vi "test_looped_handler.vi"() -> ()   [LabVIEW 2025]
uses:
  SLM parameters cluster.ctl
  <userlib>/HOLOEYE SLM Display SDK 4.1.0/types/heds_required_sdk_version_typedef.ctl
  channel parameters cluster.ctl
  <vilib>/Utility/error.llb/DialogType.ctl
  <vilib>/DAQmx/write.llb/DAQmx Write (Analog 1D Wfm NChan NSamp).vi
  <vilib>/DAQmx/write.llb/DAQmx Write (Analog 1D DBL NChan 1Samp).vi
  <vilib>/DAQmx/read.llb/DAQmx Read (Counter U32 1Chan 1Samp).vi
  <vilib>/DAQmx/read.llb/DAQmx Read (Analog Wfm 1Chan NSamp).vi
  <vilib>/Utility/config.llb/Read Key (U32).vi
  <vilib>/Utility/config.llb/Read Key (Path).vi
  <vilib>/DAQmx/miscellaneous.llb/DAQmx Fill In Error Info.vi
  <vilib>/DAQmx/create/channels.llb/DAQmx Create Channel (CI-Count Edges).vi
  <vilib>/DAQmx/configure/trigger.llb/DAQmx Start Trigger (Digital Edge).vi
  <vilib>/DAQmx/create/channels.llb/DAQmx Create Channel (CO-Pulse Generation-Time).vi
  <vilib>/DAQmx/configure/events/hardwareSignals.llb/DAQmx Export Signal (Most Signals).vi
  <resource>/dialog/BookmarkManager/managers/Default/support/User Event - Stop/BMark_User Event - Stop.lvlib
  <vilib>/Utility/config.llb/NI_LVConfig.lvlib
  <resource>/objmgr/daqmx.rc
panel:
  out "Trial progess slide":u8(slide) caption="trials" scale=0.0..5.0
  in  "Acquire time block":bool
  out "SLM image":picture
  in  "File prefix":string
  in  "Begin Experiment":bool caption="Begin experiment"
  in  "Save directory":path=path "D:/KinetixTest/SS_test"
  in  "# Trials":u32=1 caption="trials" min=1 step=1
  in  "Trial Time":dbl=1.0 caption="s" min=0.1 max=60.0 format="%#_2g"
  in  "slow camera frequency":u16(ring)=10 caption="Hz" items=["10"=10, "20"=20, "50"=50]
  in  "scan/fast camera frequency":u16(ring)=100 caption="Hz" items=["20"=20, "100"=100, "800"=800]
  in  "Pulse Duty Cycle":dbl=50.0 caption="%" min=1.0 max=100.0 step=0.1
  in  "Pulse 470":bool
  in  "Dichroic/dual imaging":bool
  out "SLM connected":bool
  in  "Connect SLM":bool
  in  "SLM default":bool
  in  "Load SLM image":bool
  in  "Create SLM image":bool
  in  "470 nm LED control":dbl(slide) step=1.0 scale=0.0..100.0 scale format="%#_3g"
  in  "594 nm laser control":dbl(slide) step=1.0 scale=0.0..100.0 scale format="%#_3g"
  in  "Run time":i32 caption="s" min=0
  in  "Run Live":bool caption="Run live"
  in  "Galvo voltage":dbl=1.0 caption="V" min=0.1 max=1.8 format="%#_2g"
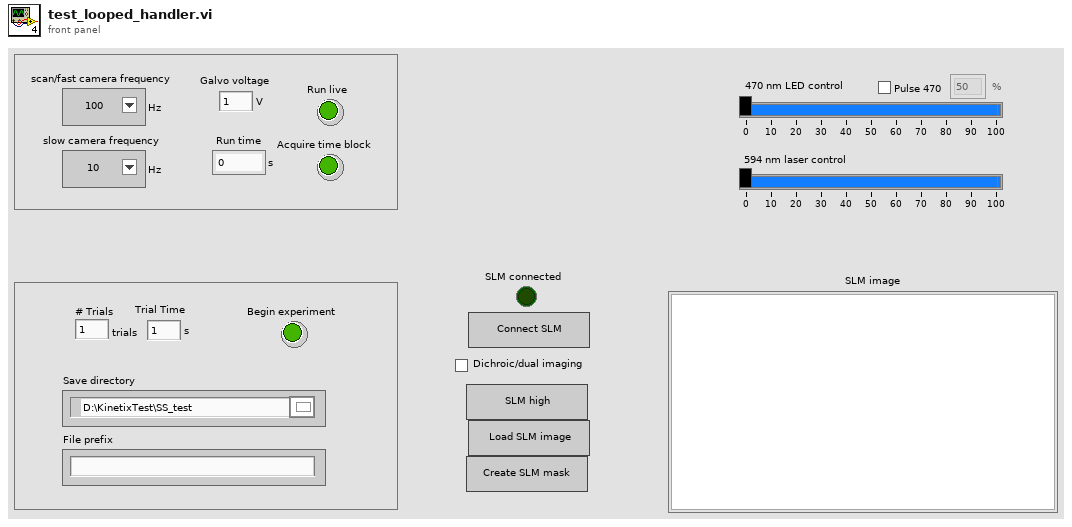
[diagram p1: front panel]
types:
  T1 = typedef "All Message Queues_TICO behavior.ctl" = cluster{"DAQ":refnum<queue>, "Acquisition":refnum<queue>, "Kinetix":refnum<queue>, "ThorCam":refnum<queue>, "SLM":refnum<queue>, "stop":refnum<queue>, " UI":refnum<queue>}
  T2 = typedef "SLM parameters cluster.ctl" = cluster{"SLM cols":u32, "SLM rows":u32, " camera image rows":u32, "camera image cols":u32, "high image (no DM)":path, "low image (no DM)":path, "high image (DM)":path, "low image (DM)":path}
  T3 = typedef "heds_required_sdk_version_typedef.ctl" = cluster{"Major Version Number":i32, "Minor Version Number":i32}
  T4 = typedef "NI_LVConfig.lvlib/Config Data RefNum.ctl" = refnum<k1>
  T5 = typedef "heds_slm_id_typedef.ctl" = cluster{"slmwindow_id":u32, "slmscreen_id":u32}
  T6 = enum8{"Enabled", "Disabled", "Disabled and Grayed Out"}
  T7 = typedef "IMAQ Image.ctl" = refnum<image>
  T8 = typedef "channel parameters cluster.ctl" = cluster{"voltage":dbl, "frequency":dbl, "duty cycle":dbl, "sample rate":dbl}
  T9 = cluster{"shutter trigger":refnum<k21>, "galvo control":refnum<k21>, "Kinetix trigger":refnum<k21>, "Kinetix readout":refnum<k21>, "Zelux trigger":refnum<k21>, "Zelux readout":refnum<k21>}
  T10 = typedef "DialogType.ctl" = u16
  T11 = enum16{"open", "open or create", "create or replace", "create", "open (read-only)"}
  T12 = typedef "Camera Description.ctl" = cluster{"Serial Number":string, "Chip Name":string, "Sensor Width":u32, "Sensor Height":u32, "Firmware version":string, "Interface":string, "Part Number":string, "Product Name":string}
  T13 = cluster{"Camera 0 Name ":string, "Camera Description":T12}
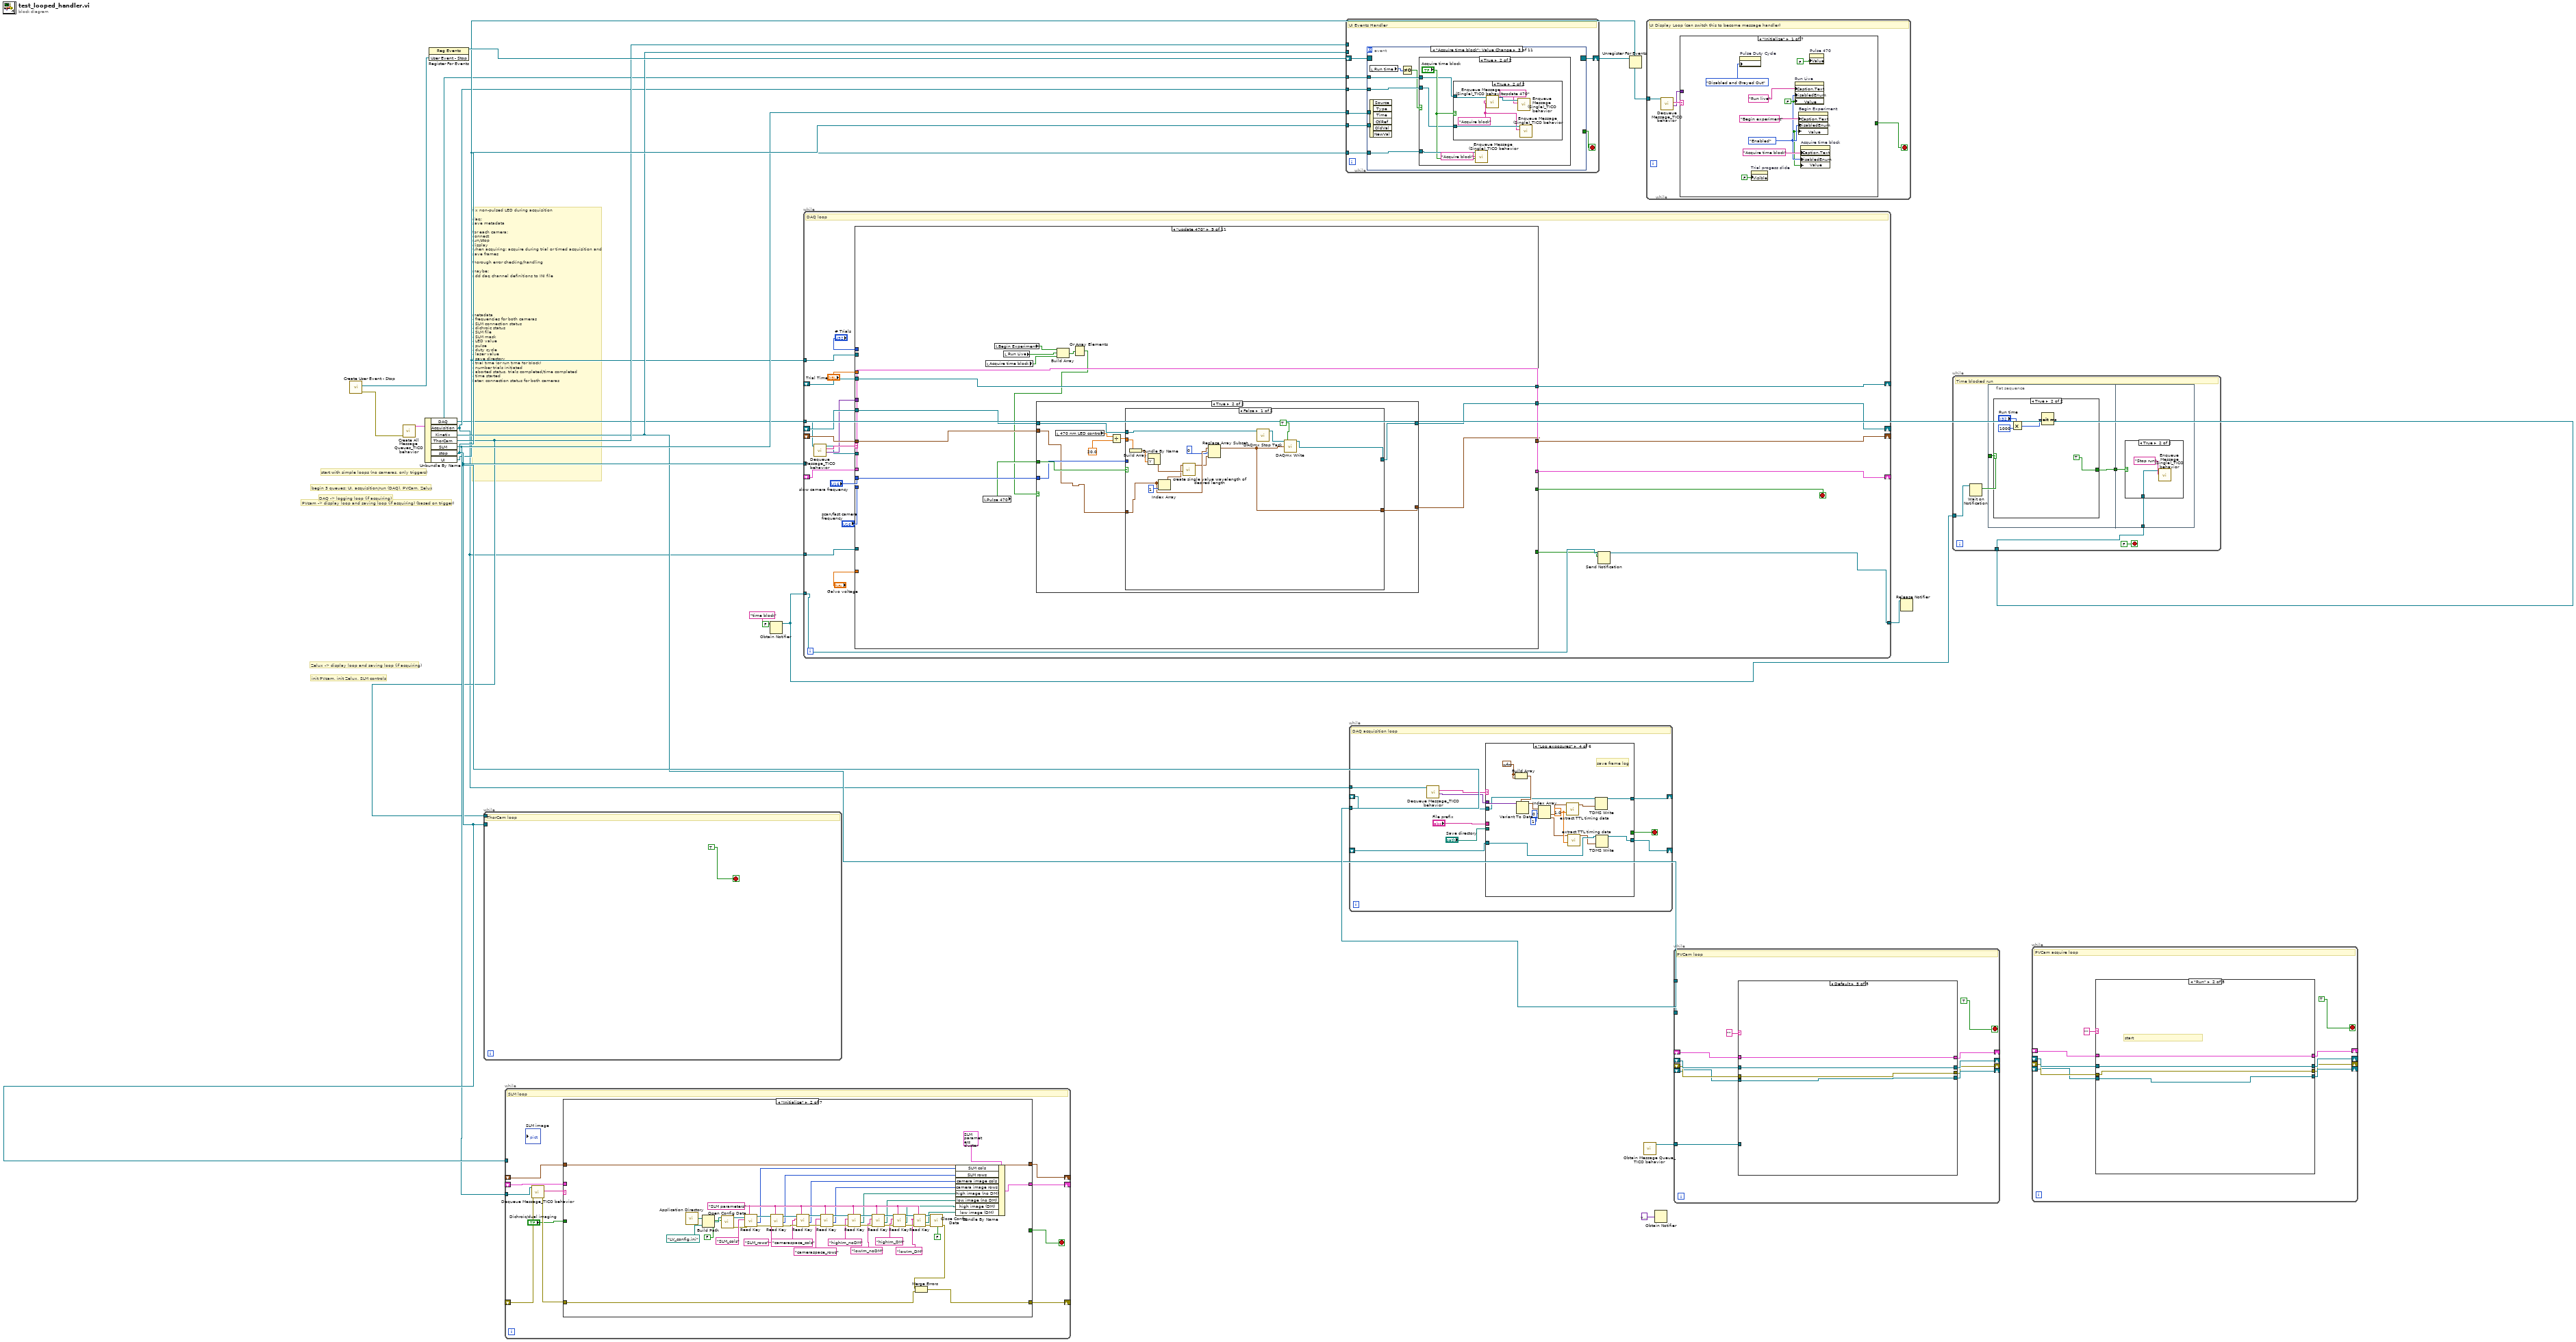
[diagram p0: block diagram]
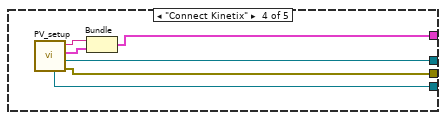
[diagram p4: hidden frame]
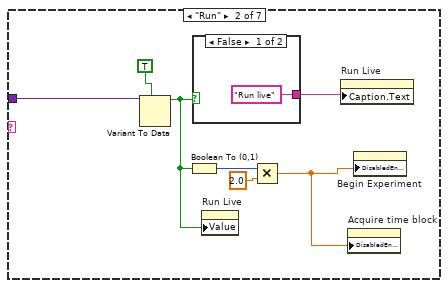
[diagram p8: hidden frame]
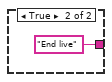
[diagram p9: hidden frame]
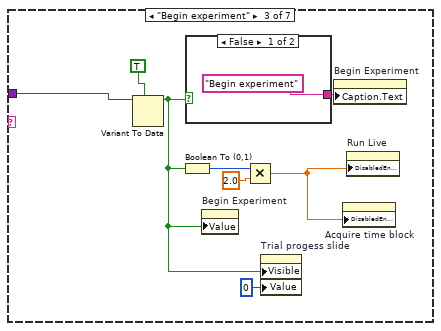
[diagram p10: hidden frame]
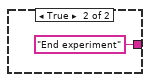
[diagram p11: hidden frame]
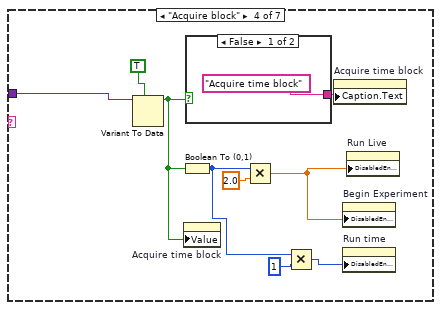
[diagram p12: hidden frame]
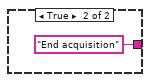
[diagram p13: hidden frame]
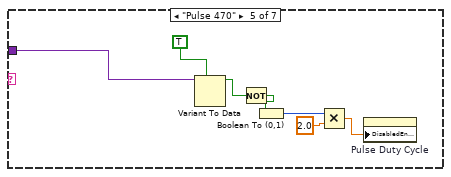
[diagram p14: hidden frame]
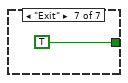
[diagram p16: hidden frame]
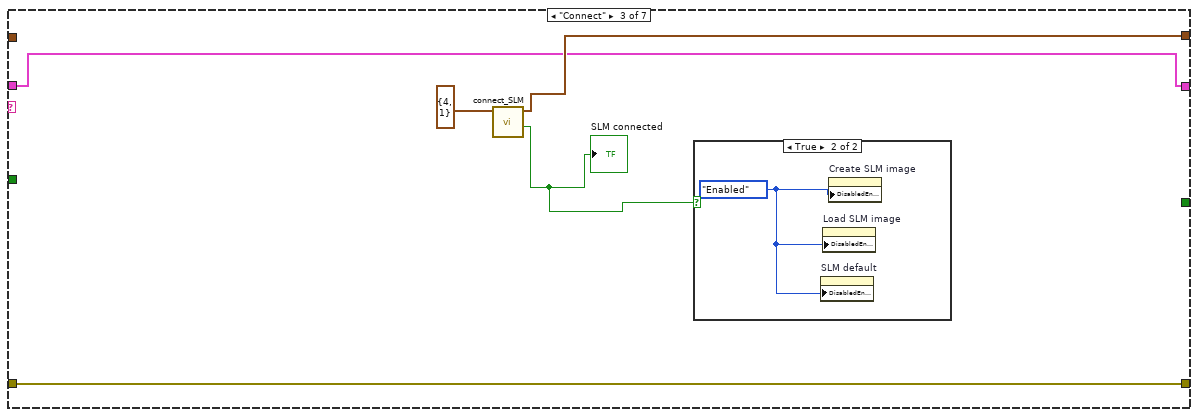
[diagram p18: hidden frame]
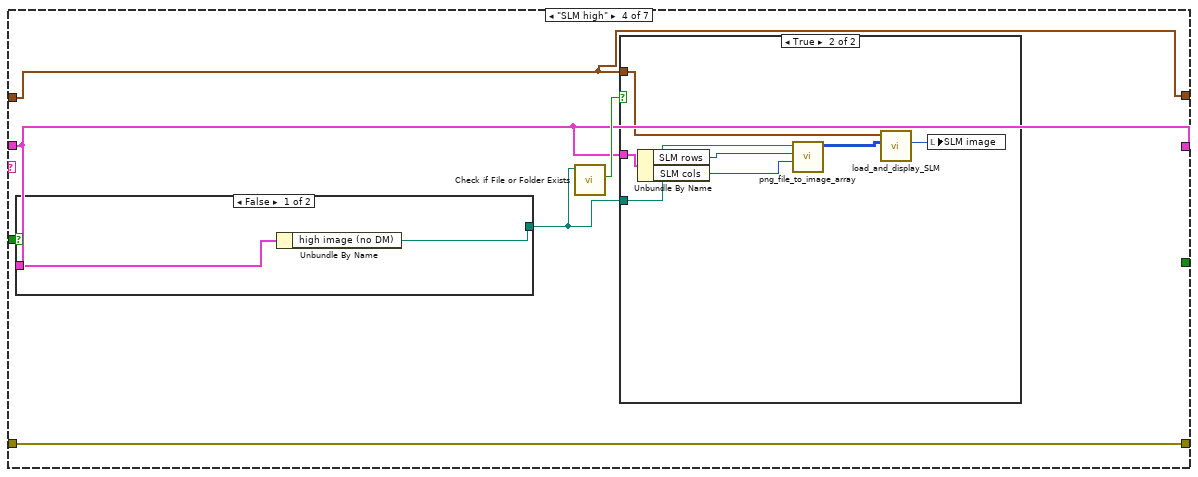
[diagram p20: hidden frame]
diagram:
  # "fix non-pulsed LED during acquisition\n\ndaq:\nsave metadata\n\nfor each camera:\nconnect\nrun/stop\ndisplay\nwhen acquiring: acquire during trial or timed acquisition and \nsave frames\n\nthorough error checking/handling\n\nmaybe:\nadd daq channel definitions to INI file\n\n\n\n\n\n\n\n\nmetadata\n- frequencies for both cameras\n- SLM connection status\n- dichroic status\n- SLM file\n- SLM mask\n- LED value\n- pulse\n- duty cycle\n- laser value\n- save directory\n- trial time (or run time for block)\n- number trials initiated\n- aborted status, trials completed/time completed \n- time started\nLater: connection status for both cameras"
  # "start with simple loops (no cameras, only triggers)"
  # "init PVcam, init Zelux, SLM controls"
  # "Zelux -> display loop and saving loop (if acquiring)"
  # "PVcam -> display loop and saving loop (if acquiring) (based on trigger)"
  # "DAQ -> logging loop (if acquiring)"
  # "begin 3 queues: UI, acquisition/run (DAQ), PVCam, Zelux"
  n1 = call <resource>:"Create User Event - Stop.vi"() -> ("error out"=w17:errorcluster, "User Event - Stop"=w16:refnum<user-event>)  [unwired: 10 in]
  n2 = call "Create All Message Queues_TICO behavior.vi"("error in (no error)"=w17) -> ("Message Queues out"=w18:T1)  [unwired: 9 in, 1 out]
  n3 = Unbundle By Name(w18) -> ("DAQ"=w3:refnum<queue>, "Acquisition"=w4:refnum<queue>, "Kinetix"=w10:refnum<queue>, "ThorCam"=w11:refnum<queue>, "SLM"=w12:refnum<queue>, "stop"=w13:refnum<queue>, "UI"=w9:refnum<queue>)
  n4 = register-events(w16) -> (reference out=w15:refnum<event-registration>)  [unwired: 2 in, 1 out]
  n5 = while {
    tunnel: w11 -> [_]
    tunnel: w13 -> [_]
    stop <- TRUE stop-if-true
    # "ThorCam loop"
  }
  n6 = while {
    tunnel: w12 -> [w27]
    tunnel: w13 -> [_]
    shift-right: [w29] -> _
    shift-left: _ -> [w28]
    shift-right: [w24] -> _
    shift-left: _ -> [w26]
    shift-right: [w22] -> _
    shift-left: _ -> [w21]
    stop <- w23 stop-if-true
    # "SLM loop"
    n7 = call "Dequeue Message_TICO behavior.vi"("error in (no error)"=w26, "Message Queue"=w27) -> ("error out"=w25:errorcluster, "Message"=w30:string)  [unwired: 6 in, 2 out]
    n8 = case shown="\"Initialize\"" w30 {
      tunnel: [w31 w79 w82 w88 w109 w123 w163] -> w29
      tunnel: w28 -> [w31 w79 _ w88 w109 w123 w163]
      tunnel: w25 -> [w32 w70 w81 w91 w108 w120 w162]
      tunnel: [w32 w71 w81 w91 w108 w120 w161] -> w24
      tunnel: [_ _ _ _ _ _ TRUE] -> w23
      tunnel: [w33 w34 w80 w86 w110 w119 w160] -> w22
      tunnel: w21 -> [w33 _ w80 w86 w110 w119 w160]
      tunnel: "Dichroic/dual imaging" -> [_ _ _ w87 _ w137 _]
      frame Default {
      }
      frame "Initialize" {
        w60 = "SLM parameters" ("section")
        n9 = call <vilib>:"Application Directory.vi"() -> ("Application Directory"=w77:path)
        n10 = Build Path(base path=w77, name or relative path=path "LV_config.ini" ("default name")) -> (appended path=w76:path)
        n11 = call <vilib>:"Open Config Data.vi"("create file if necessary (T)"=FALSE, "configuration file path"=w76) -> ("error out"=w72:errorcluster, "refnum"=w74:T4)  [unwired: 7 in, 1 out]
        n12 = call-poly <vilib>:"Read Key.vi"("section"=w60, "error in (no error)"=w72, "key"="SLM_cols", "refnum"=w74) -> ("error out"=w69:errorcluster, "value"=w42:u32, "refnum out"=w68:T4)  [unwired: 4 in, 1 out]
        n13 = call-poly <vilib>:"Read Key.vi"("section"=w60, "error in (no error)"=w69, "key"="SLM_rows", "refnum"=w68) -> ("error out"=w61:errorcluster, "value"=w41:u32, "refnum out"=w59:T4)  [unwired: 4 in, 1 out]
        n14 = call-poly <vilib>:"Read Key.vi"("section"=w60, "error in (no error)"=w61, "key"="cameraspace_cols", "refnum"=w59) -> ("error out"=w62:errorcluster, "value"=w40:u32, "refnum out"=w58:T4)  [unwired: 4 in, 1 out]
        n15 = call-poly <vilib>:"Read Key.vi"("section"=w60, "error in (no error)"=w62, "key"="cameraspace_rows", "refnum"=w58) -> ("error out"=w63:errorcluster, "value"=w39:u32, "refnum out"=w57:T4)  [unwired: 4 in, 1 out]
        n16 = call-poly <vilib>:"Read Key.vi"("section"=w60, "error in (no error)"=w63, "key"="highIm_noDM", "refnum"=w57) -> ("error out"=w64:errorcluster, "value"=w38:path, "refnum out"=w56:T4)  [unwired: 4 in, 1 out]
        n17 = call-poly <vilib>:"Read Key.vi"("section"=w60, "error in (no error)"=w64, "key"="lowIm_noDM", "refnum"=w56) -> ("error out"=w65:errorcluster, "value"=w37:path, "refnum out"=w55:T4)  [unwired: 4 in, 1 out]
        n18 = call-poly <vilib>:"Read Key.vi"("section"=w60, "error in (no error)"=w65, "key"="highIm_DM", "refnum"=w55) -> ("error out"=w66:errorcluster, "value"=w36:path, "refnum out"=w54:T4)  [unwired: 4 in, 1 out]
        n19 = call-poly <vilib>:"Read Key.vi"("section"=w60, "error in (no error)"=w66, "key"="lowIm_DM", "refnum"=w54) -> ("error out"=w53:errorcluster, "value"=w35:path, "refnum out"=w52:T4)  [unwired: 4 in, 1 out]
        n20 = call <vilib>:"Close Config Data.vi"("error in (no error)"=w53, "write file if changed (T)"=FALSE, "refnum"=w52) -> ("error out"=w50:errorcluster)  [unwired: 8 out]
        n21 = Merge Errors(w50, w70) -> (w71:errorcluster)
        n22 = Bundle By Name(cluster=T2 {"SLM cols"=0, "SLM rows"=0, " camera image rows"=0, "camera image cols"=0, "high image (no DM)"=path "", "low image (no DM)"=path "", "high image (DM)"=path "", "low image (DM)"=path ""} ("input cluster"), "SLM cols"=w42, "SLM rows"=w41, "camera image cols"=w40, "camera image rows"=w39, "high image (no DM)"=w38, "low image (no DM)"=w37, "high image (DM)"=w36, "low image (DM)"=w35) -> (w34:T2)
      }
      frame "Connect" {
        n23 = call "connect_SLM.vi"("Required SDK version"=T3 {"Major Version Number"=4, "Minor Version Number"=1}) -> ("SLM connected"=w83:bool, "SLM ID"=w82:T5)  [unwired: 9 in]
        "SLM connected" <- w83
        n24 = case shown="True" w83 {
          frame False {
          }
          frame True {
            w85 = T6."Enabled" ("Disabled")
            n25 = property on="SLM default" class="Bool"("DisabledEnum"=w85) -> ()  [unwired: 2 in, 2 out]
            n26 = property on="Load SLM image" class="Bool"("DisabledEnum"=w85) -> ()  [unwired: 2 in, 2 out]
            n27 = property on="Create SLM image" class="Bool"("DisabledEnum"=w85) -> ()  [unwired: 2 in, 2 out]
          }
        }
      }
      frame "SLM high" {
        n28 = case shown="False" w87 {
          tunnel: [w92 w94] -> w90
          tunnel: w86 -> [w93 w95]
          frame False {
            n29 = Unbundle By Name(w93) -> ("high image (no DM)"=w92:path)
          }
          frame True {
            n30 = Unbundle By Name(w95) -> ("high image (DM)"=w94:path)
          }
        }
        n31 = call <vilib>:"Check if File or Folder Exists.vi"("path"=w90) -> ("file or folder exists?"=w89:bool)  [unwired: 8 in, 2 out]
        n32 = case shown="True" w89 {
          tunnel: w90 -> [_ w102]
          tunnel: w88 -> [_ w99]
          tunnel: w86 -> [_ w98]
          frame False {
          }
          frame True {
            n33 = Unbundle By Name(w98) -> ("SLM rows"=w97:u32, "SLM cols"=w96:u32)
            n34 = call "png_file_to_image_array.vi"("dimension size 2"=w96, "dimension size 1"=w97, "path to PNG file"=w102) -> ("output array"=w101:u8[][])  [unwired: 8 in]
            n35 = call "load_and_display_SLM.vi"("Image Data"=w101, "SLM ID"=w99) -> ("2D Picture"=w100:picture)  [unwired: 8 in, 1 out]
            n36 = local write "SLM image"(w100) -> ()
          }
        }
      }
      frame "Load image" {
        n37 = local read "Save directory"() -> (w107:path)
        n38 = call "IMAQ Load Image Dialog"("Pattern"="SLM_pattern_*.png*" ("pattern (all files)"), "Multiple Files? (No)"=FALSE, "Start Path"=w107) -> ("Path"=w104:path)  [unwired: 6 in, 2 out]
        n39 = call <vilib>:"Check if File or Folder Exists.vi"("path"=w104) -> ("file or folder exists?"=w111:bool, "dup path"=w103:path)  [unwired: 8 in, 1 out]
        n40 = case shown="True" w111 {
          tunnel: w109 -> [_ w117]
          tunnel: w110 -> [_ w116]
          tunnel: w103 -> [_ w112]
          frame False {
          }
          frame True {
            n41 = Unbundle By Name(w116) -> ("SLM rows"=w115:u32, "SLM cols"=w114:u32)
            n42 = call "png_file_to_image_array.vi"("dimension size 2"=w114, "dimension size 1"=w115, "path to PNG file"=w112) -> ("output array"=w118:u8[][])  [unwired: 8 in]
            n43 = call "load_and_display_SLM.vi"("Image Data"=w118, "SLM ID"=w117) -> ("2D Picture"=w113:picture)  [unwired: 8 in, 1 out]
            n44 = local write "SLM image"(w113) -> ()
          }
        }
      }
      frame "Create mask" {
        n45 = local read "Save directory"() -> (w152:path)
        n46 = Unbundle By Name(w119) -> ("camera image rows"=w143:u32, "camera image cols"=w142:u32, "SLM rows"=w139:u32, "SLM cols"=w140:u32)
        n47 = call "IMAQ Load Image Dialog"("Pattern"="*.tif*" ("pattern (all files)"), "Multiple Files? (No)"=FALSE, "Start Path"=w152) -> ("Path"=w153:path)  [unwired: 6 in, 2 out]
        n48 = call "create ROIs GUI.vi"("Mask high value (default 255)"=sgl 255.0, "TIFF path"=w153) -> ("error out"=w148:errorcluster, "ROI mask image"=w147:T7)  [unwired: 8 in]
        n49 = case shown="False" w137 {
          tunnel: w119 -> [w156 w159]
          tunnel: [w155 w158] -> w136
          tunnel: [w154 w157] -> w135
          frame False {
            n50 = Unbundle By Name(w156) -> ("high image (no DM)"=w155:path, "low image (no DM)"=w154:path)
          }
          frame True {
            n51 = Unbundle By Name(w159) -> ("high image (DM)"=w158:path, "low image (DM)"=w157:path)
          }
        }
        n52 = call "IMAQ GetImageSize"("Image"=w147) -> ("Y Resolution"=w145:i32, "X Resolution"=w146:i32)  [unwired: 3 in, 1 out]
        n53 = call "crop_image_to_SLM_size.vi"("Y max"=w142, "X max"=w143, "error in (no error)"=w148, "Y size"=w145, "X size"=w146, "Image Src"=w147) -> ("error out"=w141:errorcluster, "Image Dst Out"=w144:T7)  [unwired: 4 in]
        n54 = call "resize camera space image to SLM space.vi"("Y SLM"=w139, "X SLM"=w140, "error in (no error)"=w141, "Y camera"=w142, "X camera"=w143, "original image"=w144) -> ("Resized image"=w138:T7)  [unwired: 4 in, 1 out]
        n55 = call "create SLM image from mask.vi"("low image path"=w135, "high image path"=w136, "Mask"=w138) -> ("Image Pixels (U8)"=w124:u8[][], "Final image"=w126:T7)  [unwired: 7 in]
        n56 = local read "File prefix"() -> (w121:string)
        n57 = local read "Save directory"() -> (w122:path)
        n58 = Format Date/Time String(time format string (%c)="%Y%m%d_%H%M%S.png") -> (date/time string=w134:string)  [unwired: 2 in]
        n59 = Concatenate Strings("SLM_pattern_" ("string"), w121, w134) -> (w133:string)
        n60 = call "load_and_display_SLM.vi"("Image Data"=w124, "SLM ID"=w123) -> ("2D Picture"=w125:picture)  [unwired: 8 in, 1 out]
        n61 = String To Path(string=w133) -> (path=w132:path)
        n62 = local write "SLM image"(w125) -> ()
        n63 = Build Path(base path=w122, name or relative path=w132) -> (appended path=w131:path)
        n64 = call-poly "IMAQ Write File 2"("Use bit depth? (false)"=TRUE, "Image Quality"=u32 1000, "File Path"=w131, "Image"=w126) -> ()  [unwired: 6 in, 2 out]
      }
      frame "Stop" {
        n65 = call <userlib>:"heds_close.vi"("error in (no error)"=w162) -> ("error out"=w161:errorcluster)  [unwired: 10 in]
      }
    }
  }
  n66 = Obtain Notifier(name (unnamed)="time block", notification data type=FALSE) -> (notifier out=w6:refnum<notifier>)  [unwired: 2 in, 2 out]
  n67 = while {
    tunnel: w3 -> [w170]
    tunnel: w13 -> [_]
    shift-right: [w184] -> _
    shift-left: _ -> [w183]
    shift-right: [w182] -> _
    shift-left: _ -> [w181]
    shift-right: [w180] -> _
    shift-left: _ -> [w179]
    tunnel: w9 -> [w176]
    tunnel: w6 -> [w174]
    tunnel: [w175] -> w7
    shift-right: [w172] -> _
    shift-left: _ -> [w171]
    tunnel: w4 -> [w168]
    stop <- w178 stop-if-true
    # "DAQ loop"
    n68 = call "Dequeue Message_TICO behavior.vi"("Message Queue"=w170) -> ("Message Data"=w166:variant, "Message"=w187:string, "dup Message Queue"=w165:refnum<queue>)  [unwired: 7 in, 1 out]
    n69 = case shown="\"update 470\"" w187 {
      selector: w187 -> [_ _ _ w264 _ _ _ _ _ _ _]
      tunnel: "scan/fast camera frequency" -> [_ w222 _ w336 _ _ _ _ _ _ _]
      tunnel: "slow camera frequency" -> [_ w223 _ w335 _ _ _ _ w513 _ _]
      tunnel: [w198 w205 w236 w332 w374 w423 w489 w499 w515 w566 w571] -> w184
      tunnel: w183 -> [_ w205 w255 w279 w374 w422 w489 w500 w516 w566 w571]
      tunnel: [w189 w224 w226 w334 w375 w416 w488 w491 w512 w565 w570] -> w182
      tunnel: w181 -> [_ w224 w229 w334 w375 w413 w488 w494 w514 w565 w570]
      tunnel: [w201 w220 T9 {"shutter trigger"="", "galvo control"="", "Kinetix trigger"="", "Kinetix readout"="", "Zelux trigger"="", "Zelux readout"=""} ("tasks cluster") w283 w372 T9 {"shutter trigger"="", "galvo control"="", "Kinetix trigger"="", "Kinetix readout"="", "Zelux trigger"="", "Zelux readout"=""} ("tasks cluster") w463 w502 w517 w564 w569] -> w180
      tunnel: w179 -> [w201 _ w254 _ w373 w457 w464 w502 w517 w564 w569]
      tunnel: [_ _ FALSE _ _ _ _ _ _ _ TRUE] -> w178
      tunnel: "Galvo voltage" -> [_ w209 _ w297 _ _ _ _ _ _ _]
      tunnel: [_ w203 _ _ _ _ _ _ _ _ _] -> w167
      tunnel: w176 -> [_ _ w232 _ _ w408 _ _ _ _ _]
      tunnel: "Trial Time" -> [_ _ _ w266 w368 _ _ _ _ _ _]
      tunnel: [w188 w202 refnum<k21> refnum ("task out") w282 w363 refnum<k21> refnum ("task out") w465 w490 w510 w563 w567] -> w172
      tunnel: w171 -> [w188 w202 _ _ w382 w431 w465 w490 w510 w563 w567]
      tunnel: w165 -> [_ _ _ w263 w381 w403 w487 _ _ _ _]
      tunnel: "# Trials" -> [_ _ _ w258 w362 _ _ _ _ _ _]
      tunnel: w168 -> [_ _ _ w281 w378 w430 _ _ _ _ _]
      tunnel: w166 -> [_ _ _ _ w364 _ _ _ _ _ _]
      frame "Initialize" {
        # "start tasks for LED and laser"
        n70 = call "init_lasers.vi"("488 pulsed"=FALSE, "594 nm voltage"=0.0, "488 nm channel parameters"=T8 {"voltage"=0.0, "frequency"=0.0, "duty cycle"=0.0, "sample rate"=1000.0}) -> ("current data"=w197:cluster{"[0]":dbl, "[1]":dbl}, "task out"=w198:refnum<k21>)  [unwired: 6 in, 1 out]
        n71 = Unbundle(w197) -> ("[0]"=w196:dbl, "[1]"=w193:dbl)
        n72 = Build Array(w196) -> (w195:dbl[])
        n73 = Build Array(w193) -> (w194:dbl[])
        n74 = Bundle By Name("Y"=w195) -> (w191:waveform(dbl))  [unwired: 1 in]
        n75 = Bundle By Name("Y"=w194) -> (w190:waveform(dbl))  [unwired: 1 in]
        n76 = Build Array(w191, w190) -> (w189:waveform(dbl)[])
      }
      frame "Run" {
        n77 = call "init_DAQ_cluster.vi"("Slow/Zelux frame frequency"=w223, "Fast/Kinetix frame frequency"=w222) -> ("tasks cluster"=w221:T9)  [unwired: 8 in, 1 out]
        n78 = Unbundle By Name(w221) -> ("shutter trigger"=w219:refnum<k21>, "galvo control"=w211:refnum<k21>, "Kinetix trigger"=w213:refnum<k21>, "Zelux trigger"=w207:refnum<k21>)
        n79 = property class="DAQmx Channel"(reference=w213) -> ("CO.Pulse.Freq"=w212:dbl)  [unwired: 1 in, 2 out]
        n80 = property class="DAQmx Timing"(reference=w211) -> ("SampClk.Rate"=w210:dbl)  [unwired: 1 in, 2 out]
        n81 = call "galvo_triangle_wave.vi"("final frequency"=w212, "amplitude"=w209, "sample rate"=w210) -> ("waveform array out"=w216:waveform(dbl)[])  [unwired: 8 in]
        n82 = call-poly <vilib>:"DAQmx Write.vi"("task/channels in"=w211, "data"=w216) -> ("task out"=w215:refnum<k21>, "error out"=w214:errorcluster)  [unwired: 11 in, 1 out]
        n83 = call <vilib>:"DAQmx Start Task.vi"("task/channels in"=w219) -> ("task out"=w208:refnum<k21>)  [unwired: 13 in, 1 out]
        n84 = call <vilib>:"DAQmx Start Task.vi"("task/channels in"=w213) -> ("task out"=w218:refnum<k21>)  [unwired: 13 in, 1 out]
        n85 = call <vilib>:"DAQmx Start Task.vi"("task/channels in"=w215, "error in"=w214) -> ("task out"=w217:refnum<k21>)  [unwired: 12 in, 1 out]
        n86 = call <vilib>:"DAQmx Start Task.vi"("task/channels in"=w207) -> ("task out"=w206:refnum<k21>)  [unwired: 13 in, 1 out]
        n87 = Bundle By Name(cluster=w221, "shutter trigger"=w208, "galvo control"=w217, "Kinetix trigger"=w218, "Kinetix readout"=w206) -> (w220:T9)
        n88 = local read "Run time"() -> (w204:i32)
        n89 = Not Equal To 0?(x=w204) -> (x != 0?=w203:bool)
      }
      frame "Stop run" {
        (unwired) 1 ("index")
        w240 = T10 0 items=["no dialog", "OK message", "continue or stop message", "OK message + warnings", "continue/stop + warnings"] ("type of dialog (OK msg:1)")
        n90 = Unbundle By Name(w254) -> ("shutter trigger"=w237:refnum<k21>, "galvo control"=w252:refnum<k21>, "Kinetix trigger"=w250:refnum<k21>, "Zelux trigger"=w246:refnum<k21>)
        n91 = Build Array(0.0 ("data")) -> (w230:dbl[])
        n92 = Bundle By Name("Y"=w230) -> (w227:waveform(dbl))  [unwired: 1 in]
        n93 = call <vilib>:"DAQmx Stop Task.vi"("task/channels in"=w237) -> ("task out"=w239:refnum<k21>, "error out"=w238:errorcluster)  [unwired: 13 in]
        n94 = call <vilib>:"DAQmx Stop Task.vi"("task/channels in"=w252) -> ("task out"=w251:refnum<k21>, "error out"=w249:errorcluster)  [unwired: 13 in]
        n95 = call <vilib>:"DAQmx Stop Task.vi"("task/channels in"=w246) -> ("task out"=w245:refnum<k21>, "error out"=w244:errorcluster)  [unwired: 13 in]
        n96 = call <vilib>:"DAQmx Stop Task.vi"("task/channels in"=w250) -> ("task out"=w248:refnum<k21>, "error out"=w247:errorcluster)  [unwired: 13 in]
        n97 = Replace Array Subset(array=w229, new element=w227, index=0) -> (w226:waveform(dbl)[])
        n98 = call <vilib>:"DAQmx Clear Task.vi"("task in"=w239, "error in"=w238) -> ("error out"=w243:errorcluster)  [unwired: 13 in]
        n99 = call <vilib>:"DAQmx Clear Task.vi"("task in"=w245, "error in"=w244) -> ("error out"=w242:errorcluster)  [unwired: 13 in]
        n100 = call "galvo_recenter.vi"("error in"=w249, "task/channels in"=w251) -> ()  [unwired: 10 in]
        n101 = call <vilib>:"DAQmx Clear Task.vi"("task in"=w248, "error in"=w247) -> ("error out"=w241:errorcluster)  [unwired: 13 in]
        n102 = call <vilib>:"Simple Error Handler.vi"("type of dialog (OK msg:1)"=w240, "error in (no error)"=w243) -> ()  [unwired: 3 in, 5 out]
        n103 = call-poly <vilib>:"DAQmx Write.vi"("task/channels in"=w255, "auto start"=TRUE, "data"=w226) -> ("task out"=w236:refnum<k21>)  [unwired: 10 in, 2 out]
        n104 = call <vilib>:"Simple Error Handler.vi"("type of dialog (OK msg:1)"=w240, "error in (no error)"=w241) -> ()  [unwired: 3 in, 5 out]
        n105 = call <vilib>:"Simple Error Handler.vi"("type of dialog (OK msg:1)"=w240, "error in (no error)"=w242) -> ()  [unwired: 3 in, 5 out]
        n106 = call "Enqueue Message (Single)_TICO behavior.vi"("Message Data"=FALSE, "Message"="Run", "Message Queue"=w232) -> ()  [unwired: 7 in, 2 out]
      }
      frame "Acquire block", "Begin Experiment" {
        w288 = 10280 items=["Rising"=10280, "Falling"=10171] ("edge")
        w326 = 10178 items=["Finite Samples"=10178, "Continuous Samples"=10123, "Hardware Timed Single Point"=12522] ("SampQuant.SampMode")
        w328 = 10150 items=["Analog Edge"=10099, "Analog Multi Edge"=16108, "Digital Edge"=10150, "Digital Pattern"=10398, "Analog Window"=10103, "Time"=15996, "None"=10230] ("Start.TrigType")
        w286 = tag "/GalvoPMT/PFI9" ("source")
        # "min pulse width ensures proper increment/debouncing"
        n107 = case shown="\"Acquire block\"" w264 {
          tunnel: w266 -> [_ w348 w349]
          tunnel: [w345 w348 w349] -> w265
          tunnel: w258 -> [_ w347 _]
          frame "Acquire block" {
            n108 = local read "Run time"() -> (w346:i32)
            n109 = To Double Precision Float(number=w346) -> (double precision float=w345:dbl)
          }
          frame "Begin experiment" {
            n110 = property on="Trial progess slide" class="Slide (strict)"("Scale.Maximum"=w347) -> ()  [unwired: 2 in, 2 out]
          }
          frame Default {
          }
        }
        n111 = call "init_DAQ_cluster.vi"("Sample rate"=100000.0, "Slow/Zelux frame frequency"=w335, "Fast/Kinetix frame frequency"=w336) -> ("tasks cluster"=w314:T9)  [unwired: 7 in, 1 out]
        n112 = call <vilib>:"DAQmx Stop Task.vi"("task/channels in"=w279) -> ("task out"=w278:refnum<k21>, "error out"=w257:errorcluster)  [unwired: 13 in]
        n113 = property class="DAQmx Timing"(reference=w278, error in=w257) -> (reference out=w323:refnum<k21>, "SampClk.Rate"=w322:dbl)  [unwired: 1 out]
        n114 = Unbundle By Name(w314) -> ("shutter trigger"=w321:refnum<k21>, "galvo control"=w274:refnum<k21>, "Kinetix trigger"=w270:refnum<k21>, "Kinetix readout"=w333:refnum<k21>, "Zelux trigger"=w267:refnum<k21>, "Zelux readout"=w271:refnum<k21>)
        n115 = property class="DAQmx Timing"(reference=w274) -> ("SampClk.Rate"=w295:dbl)  [unwired: 1 in, 2 out]
        n116 = property class="DAQmx Channel"(reference=w270) -> ("CO.Pulse.Freq"=w294:dbl)  [unwired: 1 in, 2 out]
        n117 = property class="DAQmx Channel"(reference=w267) -> ("CO.Pulse.Freq"=w269:dbl)  [unwired: 1 in, 2 out]
        n118 = Divide(x=1.0, y=w265) -> (x/y=w276:dbl)
        n119 = call "galvo_triangle_wave.vi"("trial seconds"=w265, "final frequency"=w294, "amplitude"=w297, "sample rate"=w295) -> ("waveform array out"=w298:waveform(dbl)[])  [unwired: 7 in]
        n120 = Multiply(x=w269, y=w265) -> (x*y=w268:dbl)
        n121 = Multiply(x=w322, y=w265) -> (x*y=w325:dbl)
        n122 = Multiply(x=w295, y=w265) -> (x*y=w272:dbl)
        n123 = Multiply(x=w294, y=w265) -> (x*y=w273:dbl)
        n124 = property class="DAQmx Channel"(reference=w321, "CO.Pulse.Freq"=w276) -> (reference out=w320:refnum<k21>, error out=w318:errorcluster)  [unwired: 1 in]
        n125 = call "set up centrally triggered task.vi"("SampQuant.SampPerChan"=w272, "source"=w286, "task/channels in"=w333) -> ("error out"=w301:errorcluster, "task out"=w312:refnum<k21>)  [unwired: 7 in]
        n126 = call "set up centrally triggered task.vi"("SampQuant.SampPerChan"=w273, "source"=w286, "task/channels in"=w270) -> ("error out"=w302:errorcluster, "task out"=w311:refnum<k21>)  [unwired: 7 in]
        n127 = call "set up centrally triggered task.vi"("SampQuant.SampPerChan"=w272, "source"=w286, "task/channels in"=w274) -> ("error out"=w303:errorcluster, "task out"=w304:refnum<k21>)  [unwired: 7 in]
        n128 = call "set up centrally triggered task.vi"("SampQuant.SampPerChan"=w268, "source"=w286, "task/channels in"=w267) -> ("error out"=w300:errorcluster, "task out"=w310:refnum<k21>)  [unwired: 7 in]
        n129 = call "set up centrally triggered task.vi"("SampQuant.SampPerChan"=w272, "source"=w286, "task/channels in"=w271) -> ("error out"=w299:errorcluster, "task out"=w309:refnum<k21>)  [unwired: 7 in]
        n130 = call <vilib>:"DAQmx Start Task.vi"("task/channels in"=w312, "error in"=w301) -> ("task out"=w259:refnum<k21>)  [unwired: 12 in, 1 out]
        n131 = call <vilib>:"DAQmx Start Task.vi"("task/channels in"=w310, "error in"=w300) -> ("task out"=w308:refnum<k21>)  [unwired: 12 in, 1 out]
        n132 = call <vilib>:"DAQmx Start Task.vi"("task/channels in"=w309, "error in"=w299) -> ("task out"=w260:refnum<k21>)  [unwired: 12 in, 1 out]
        n133 = property class="DAQmx Timing"(reference=w323, "Sample Quantity:Sample Mode"=w326, "SampQuant.SampPerChan"=w325) -> (reference out=w324:refnum<k21>)  [unwired: 1 in, 1 out]
        n134 = call <vilib>:"DAQmx Start Task.vi"("task/channels in"=w311, "error in"=w302) -> ("task out"=w296:refnum<k21>)  [unwired: 12 in, 1 out]
        n135 = call-poly <vilib>:"DAQmx Write.vi"("task/channels in"=w304, "data"=w298, "error in"=w303) -> ("task out"=w306:refnum<k21>, "error out"=w305:errorcluster)  [unwired: 10 in, 1 out]
        n136 = call-poly <vilib>:"DAQmx Trigger.vi"("task/channels in"=w320, "source"=w286, "error in"=w318) -> ("task out"=w319:refnum<k21>, "error out"=w317:errorcluster)  [unwired: 11 in]
        n137 = property class="DAQmx Trigger"(reference=w324, "Start.Retriggerable"=TRUE, "Start.TrigType"=w328) -> (reference out=w327:refnum<k21>)  [unwired: 1 in, 1 out]
        n138 = property class="DAQmx Trigger"(reference=w319, error in=w317, "Start.Retriggerable"=TRUE) -> (reference out=w316:refnum<k21>, error out=w315:errorcluster)
        n139 = call <vilib>:"DAQmx Start Task.vi"("task/channels in"=w306, "error in"=w305) -> ("task out"=w307:refnum<k21>)  [unwired: 12 in, 1 out]
        n140 = call "Enqueue Message (Single)_TICO behavior.vi"("Message"="Acquire experiment", "Message Queue"=w281) -> ()  [unwired: 8 in, 2 out]
        n141 = call-poly <vilib>:"DAQmx Create Virtual Channel.vi"("initial count"=u32 0, "edge"=w288, "counter"=tag "GalvoPMT/ctr2") -> ("task out"=w292:refnum<k21>, "error out"=w284:errorcluster)  [unwired: 11 in]
        n142 = call <vilib>:"DAQmx Start Task.vi"("task/channels in"=w316, "error in"=w315) -> ("task out"=w313:refnum<k21>)  [unwired: 12 in, 1 out]
        n143 = Bundle By Name(cluster=w314, "shutter trigger"=w313, "galvo control"=w307, "Kinetix trigger"=w296, "Kinetix readout"=w259, "Zelux trigger"=w308, "Zelux readout"=w260) -> (w283:T9)
        n144 = call-poly <vilib>:"DAQmx Trigger.vi"("task/channels in"=w327, "source"=w286) -> ("task out"=w331:refnum<k21>, "error out"=w330:errorcluster)  [unwired: 12 in]
        n145 = property class="DAQmx Channel"(reference=w292, error in=w284, "CI.CountEdges.Term"=w286, "CI.CountEdges.DigFltr.MinPulseWidth"=1e-06 ("DI.DigFltr.MinPulseWidth")) -> (reference out=w290:refnum<k21>, error out=w285:errorcluster)
        n146 = call <vilib>:"DAQmx Start Task.vi"("task/channels in"=w331, "error in"=w330) -> ("task out"=w332:refnum<k21>)  [unwired: 12 in, 1 out]
        n147 = case shown="\"Acquire block\"" w264 {
          tunnel: w263 -> [w340 w342 w344]
          tunnel: [w341 w342 w344] -> w262
          tunnel: ["block" _ "experiment"] -> w261
          frame "Acquire block" {
            n148 = call "Enqueue Message (Single)_TICO behavior.vi"("Message"="Trigger acquire block", "Message Queue"=w340) -> ("dup Message Queue"=w341:refnum<queue>)  [unwired: 8 in, 1 out]
          }
          frame Default {
          }
          frame "Begin experiment" {
          }
        }
        n149 = call <vilib>:"DAQmx Start Task.vi"("task/channels in"=w290, "error in"=w285) -> ("task out"=w282:refnum<k21>)  [unwired: 12 in, 1 out]
        n150 = call "Enqueue Message (Single)_TICO behavior.vi"("Message Data"=w261, "Message"="Continue experiment", "Message Queue"=w262) -> ()  [unwired: 7 in, 2 out]
      }
      frame "Continue experiment" {
        w350 = 20.0 ("timeout")
        # "must stop/restart to reset t0"
        n151 = Variant To Data(type="", Variant=w364) -> (data=w365:string)  [unwired: 1 in, 1 out]
        n152 = case shown="\"experiment\"" w365 {
          tunnel: [u32 1 w388 w391] -> w369
          tunnel: w362 -> [_ w389 w391]
          tunnel: w368 -> [_ w390 w392]
          tunnel: [w385 w390 w392] -> w367
          frame "block" {
            n153 = local read "Run time"() -> (w384:i32)
            n154 = To Double Precision Float(number=w384) -> (double precision float=w385:dbl)
          }
          frame "experiment" {
            n155 = Subtract(x=w389, y=u32 1) -> (x-y=w388:u32)
          }
          frame Default {
          }
        }
        n156 = Unbundle By Name(w373) -> ("Kinetix readout"=w380:refnum<k21>, "Zelux readout"=w379:refnum<k21>)
        n157 = call-poly <vilib>:"DAQmx Read.vi"("task/channels in"=w382) -> ("task out"=w363:refnum<k21>, "data"=w361:u32)  [unwired: 12 in, 1 out]
        "Trial progess slide" <- w361
        n158 = call-poly <vilib>:"DAQmx Read.vi"("task/channels in"=w379, "timeout"=w350) -> ("task out"=w358:refnum<k21>, "data"=w370:waveform(dbl), "error out"=w357:errorcluster)  [unwired: 11 in]
        n159 = call-poly <vilib>:"DAQmx Read.vi"("task/channels in"=w380, "timeout"=w350) -> ("task out"=w359:refnum<k21>, "data"=w371:waveform(dbl), "error out"=w360:errorcluster)  [unwired: 11 in]
        n160 = Greater Or Equal?(x=w361, y=w369) -> (x >= y?=w383:bool)
        n161 = case shown="True" w383 {
          tunnel: w367 -> [_ w398]
          tunnel: w381 -> [w395 w397]
          tunnel: w364 -> [w393 _]
          frame False {
            n162 = call "Enqueue Message (Single)_TICO behavior.vi"("Message Data"=w393, "Message"="Continue experiment", "Message Queue"=w395) -> ()  [unwired: 7 in, 2 out]
          }
          frame True {
            n163 = while {
              tunnel: [w402] -> w396
              tunnel: w398 -> [w401]
              stop <- w402 stop-if-true
              n164 = call "Elapsed Time2"("Time Target (s)"=w401) -> ("Time has Elapsed"=w402:bool)  [unwired: 11 in, 7 out]
            }
            n165 = case shown="True" w396 {
              tunnel: w397 -> [_ w399]
              frame False {
              }
              frame True {
                n166 = call "Enqueue Message (Single)_TICO behavior.vi"("Message"="Stop experiment", "Message Queue"=w399) -> ()  [unwired: 8 in, 2 out]
              }
            }
          }
        }
        n167 = call <vilib>:"DAQmx Stop Task.vi"("task/channels in"=w358, "error in"=w357) -> ("task out"=w353:refnum<k21>, "error out"=w351:errorcluster)  [unwired: 12 in]
        n168 = Build Array(w371, w370) -> (w376:waveform(dbl)[])
        n169 = call <vilib>:"DAQmx Stop Task.vi"("task/channels in"=w359, "error in"=w360) -> ("task out"=w356:refnum<k21>, "error out"=w354:errorcluster)  [unwired: 12 in]
        n170 = call <vilib>:"DAQmx Start Task.vi"("task/channels in"=w353, "error in"=w351) -> ("task out"=w352:refnum<k21>)  [unwired: 12 in, 1 out]
        n171 = call <vilib>:"DAQmx Start Task.vi"("task/channels in"=w356, "error in"=w354) -> ("task out"=w355:refnum<k21>)  [unwired: 12 in, 1 out]
        n172 = call "Enqueue Message (Single)_TICO behavior.vi"("Message Data"=w376, "Message"="log exposures", "Message Queue"=w378) -> ()  [unwired: 7 in, 2 out]
        n173 = Bundle By Name(cluster=w373, "Kinetix readout"=w355, "Zelux readout"=w352) -> (w372:T9)
      }
      frame "Stop experiment" {
        w426 = 10230 items=["Analog Edge"=10099, "Analog Multi Edge"=16108, "Digital Edge"=10150, "Digital Pattern"=10398, "Analog Window"=10103, "Time"=15996, "None"=10230] ("Start.TrigType")
        w428 = 10123 items=["Finite Samples"=10178, "Continuous Samples"=10123, "Hardware Timed Single Point"=12522] ("SampQuant.SampMode")
        w405 = T10 0 items=["no dialog", "OK message", "continue or stop message", "OK message + warnings", "continue/stop + warnings"] ("type of dialog (OK msg:1)")
        # "stops calls to continue run (with nonexistent tasks) if queue had extra calls"
        n174 = Flush Queue(queue=w403) -> ()  [unwired: 1 in, 3 out]
        n175 = call <vilib>:"DAQmx Stop Task.vi"("task/channels in"=w422) -> ("task out"=w421:refnum<k21>)  [unwired: 13 in, 1 out]
        n176 = property class="DAQmx Trigger"(reference=w421, "Start:Trigger Type"=w426, "Start.Retriggerable"=FALSE) -> (reference out=w427:refnum<k21>)  [unwired: 1 in, 1 out]
        n177 = Unbundle By Name(w457) -> ("shutter trigger"=w442:refnum<k21>, "galvo control"=w441:refnum<k21>, "Kinetix trigger"=w440:refnum<k21>, "Kinetix readout"=w404:refnum<k21>, "Zelux trigger"=w439:refnum<k21>, "Zelux readout"=w437:refnum<k21>)
        n178 = property class="DAQmx Timing"(reference=w427, "Sample Quantity:Sample Mode"=w428) -> (reference out=w424:refnum<k21>)  [unwired: 1 in, 1 out]
        n179 = Build Array(0.0 ("data")) -> (w418:dbl[])
        n180 = Index Array(array=w413, index=1) -> (element=w411:waveform(dbl))
        n181 = Bundle By Name("Y"=w418) -> (w415:waveform(dbl))  [unwired: 1 in]
        n182 = call <vilib>:"DAQmx Stop Task.vi"("task/channels in"=w442) -> ("task out"=w444:refnum<k21>, "error out"=w443:errorcluster)  [unwired: 13 in]
        n183 = call "create single value wavelength of desired length.vi"("waveform (with desired single value)"=w415, "waveform in (for length)"=w411) -> ("output waveform"=w414:waveform(dbl))  [unwired: 9 in]
        n184 = Replace Array Subset(array=w413, new element=w414, index=0) -> (w416:waveform(dbl)[])
        n185 = call <vilib>:"DAQmx Stop Task.vi"("task/channels in"=w404) -> ("task out"=w435:refnum<k21>)  [unwired: 13 in, 1 out]
        n186 = call <vilib>:"DAQmx Stop Task.vi"("task/channels in"=w441) -> ("task out"=w453:refnum<k21>, "error out"=w452:errorcluster)  [unwired: 13 in]
        n187 = call <vilib>:"DAQmx Stop Task.vi"("task/channels in"=w440) -> ("task out"=w451:refnum<k21>, "error out"=w450:errorcluster)  [unwired: 13 in]
        n188 = call <vilib>:"DAQmx Stop Task.vi"("task/channels in"=w439) -> ("task out"=w449:refnum<k21>, "error out"=w448:errorcluster)  [unwired: 13 in]
        n189 = call <vilib>:"DAQmx Stop Task.vi"("task/channels in"=w437) -> ("task out"=w438:refnum<k21>)  [unwired: 13 in, 1 out]
        n190 = call <vilib>:"DAQmx Clear Task.vi"("task in"=w444, "error in"=w443) -> ("error out"=w447:errorcluster)  [unwired: 13 in]
        n191 = call <vilib>:"DAQmx Stop Task.vi"("task/channels in"=w431) -> ("task out"=w433:refnum<k21>, "error out"=w407:errorcluster)  [unwired: 13 in]
        n192 = call <vilib>:"DAQmx Clear Task.vi"("task in"=w435) -> ("error out"=w434:errorcluster)  [unwired: 14 in]
        n193 = call <vilib>:"DAQmx Clear Task.vi"("task in"=w438) -> ("error out"=w436:errorcluster)  [unwired: 14 in]
        n194 = call "galvo_recenter.vi"("error in"=w452, "task/channels in"=w453) -> ()  [unwired: 10 in]
        n195 = call <vilib>:"DAQmx Clear Task.vi"("task in"=w451, "error in"=w450) -> ("error out"=w445:errorcluster)  [unwired: 13 in]
        n196 = call <vilib>:"DAQmx Clear Task.vi"("task in"=w449, "error in"=w448) -> ("error out"=w446:errorcluster)  [unwired: 13 in]
        n197 = call <vilib>:"Simple Error Handler.vi"("type of dialog (OK msg:1)"=w405, "error in (no error)"=w447) -> ()  [unwired: 3 in, 5 out]
        n198 = call <vilib>:"DAQmx Clear Task.vi"("task in"=w433, "error in"=w407) -> ("error out"=w432:errorcluster)  [unwired: 13 in]
        n199 = call-poly <vilib>:"DAQmx Write.vi"("task/channels in"=w424, "auto start"=TRUE, "data"=w416) -> ("task out"=w423:refnum<k21>)  [unwired: 10 in, 2 out]
        n200 = call <vilib>:"Simple Error Handler.vi"("type of dialog (OK msg:1)"=w405, "error in (no error)"=w445) -> ()  [unwired: 3 in, 5 out]
        n201 = call <vilib>:"Simple Error Handler.vi"("type of dialog (OK msg:1)"=w405, "error in (no error)"=w434) -> ()  [unwired: 3 in, 5 out]
        n202 = call <vilib>:"Simple Error Handler.vi"("type of dialog (OK msg:1)"=w405, "error in (no error)"=w436) -> ()  [unwired: 3 in, 5 out]
        n203 = call <vilib>:"Simple Error Handler.vi"("type of dialog (OK msg:1)"=w405, "error in (no error)"=w446) -> ()  [unwired: 3 in, 5 out]
        n204 = call <vilib>:"Simple Error Handler.vi"("type of dialog (OK msg:1)"=w405, "error in (no error)"=w432) -> ()  [unwired: 3 in, 5 out]
        n205 = call "Enqueue Message (Single)_TICO behavior.vi"("Message Data"=FALSE, "Message"="Begin experiment", "Message Queue"=w408) -> ()  [unwired: 7 in, 2 out]
        n206 = call "Enqueue Message (Single)_TICO behavior.vi"("Message"="end acquisition", "Message Queue"=w430) -> ()  [unwired: 8 in, 2 out]
        n207 = call "Enqueue Message (Single)_TICO behavior.vi"("Message Data"=FALSE, "Message"="Acquire block", "Message Queue"=w408) -> ()  [unwired: 7 in, 2 out]
      }
      frame "Trigger acquire block" {
        w460 = TRUE ("ReadAllAvailSamp")
        w472 = 10451 items=["Sample Clock"=10388, "Burst Handshake"=12548, "Handshake"=10389, "Implicit"=10451, "On Demand"=10390, "Change Detection"=12504, "Pipelined Sample Clock"=14668] ("SampTimingType")
        w479 = 10178 items=["Finite Samples"=10178, "Continuous Samples"=10123, "Hardware Timed Single Point"=12522] ("SampQuant.SampMode")
        w481 = 12494 items=["AI Convert Clock"=12484, "10MHz Reference Clock"=12536, "20MHz Timebase Clock"=12486, "Sample Clock"=12487, "Advance Trigger"=12488, "Reference Trigger"=12490, "Start Trigger"=12491, "Advance Complete Event"=12492, "AI Hold Complete Event"=12493, "Counter Output Event"=12494, "Change Detection Event"=12511, "Watchdog Timer Expired Event"=12512] ("signal")
        w482 = 0.001 ("high time")
        n208 = Unbundle By Name(w464) -> ("Kinetix readout"=w462:refnum<k21>, "Zelux readout"=w459:refnum<k21>)
        n209 = property class="DAQmx Read"(reference=w462, "ReadAllAvailSamp"=w460) -> (reference out=w461:refnum<k21>)  [unwired: 1 in, 1 out]
        n210 = property class="DAQmx Read"(reference=w459, "ReadAllAvailSamp"=w460) -> (reference out=w458:refnum<k21>)  [unwired: 1 in, 1 out]
        n211 = Bundle By Name(cluster=w464, "Kinetix readout"=w461, "Zelux readout"=w458) -> (w463:T9)
        n212 = call "Enqueue Message (Single)_TICO behavior.vi"("Message Data"="block" ("Message"), "Message"="continue experiment", "Message Queue"=w487) -> ()  [unwired: 7 in, 2 out]
        n213 = call-poly <vilib>:"DAQmx Create Virtual Channel.vi"("high time"=w482, "low time"=w482, "counter"=tag "GalvoPMT/ctr3") -> ("task out"=w478:refnum<k21>, "error out"=w477:errorcluster)  [unwired: 11 in]
        n214 = property class="DAQmx Timing"(reference=w478, error in=w477, "SampQuant.SampMode"=w479, "SampTimingType"=w472, "SampQuant.SampPerChan"=1.0 ("SampClk.Rate")) -> (reference out=w474:refnum<k21>, error out=w473:errorcluster)
        n215 = call-poly <vilib>:"DAQmx Export Signal.vi"("task/channels in"=w474, "signal"=w481, "output terminal"=tag "/GalvoPMT/PFI9", "error in"=w473) -> ("task out"=w470:refnum<k21>, "error out"=w469:errorcluster)  [unwired: 10 in]
        n216 = call <vilib>:"DAQmx Start Task.vi"("task/channels in"=w470, "error in"=w469) -> ("task out"=w467:refnum<k21>, "error out"=w468:errorcluster)  [unwired: 12 in]
        n217 = call <vilib>:"DAQmx Wait Until Done.vi"("task/channels in"=w467, "error in"=w468) -> ("task out"=w485:refnum<k21>, "error out"=w484:errorcluster)  [unwired: 12 in]
        n218 = call <vilib>:"DAQmx Stop Task.vi"("task/channels in"=w485, "error in"=w484) -> ("task out"=w476:refnum<k21>, "error out"=w475:errorcluster)  [unwired: 12 in]
        n219 = call <vilib>:"DAQmx Clear Task.vi"("task in"=w476, "error in"=w475) -> ()  [unwired: 13 in, 1 out]
      }
      frame "update 594" {
        n220 = local read "594 nm laser control"() -> (w504:dbl)
        n221 = Divide(x=w504, y=20.0) -> (x/y=w498:dbl)
        n222 = Index Array(array=w494) -> (element=w496:waveform(dbl))  [unwired: 1 in]
        n223 = Build Array(w498) -> (w497:dbl[])
        n224 = Bundle By Name("Y"=w497) -> (w495:waveform(dbl))  [unwired: 1 in]
        n225 = call "create single value wavelength of desired length.vi"("waveform (with desired single value)"=w495, "waveform in (for length)"=w496) -> ("output waveform"=w493:waveform(dbl))  [unwired: 9 in]
        n226 = Replace Array Subset(array=w494, new element=w493, index=1) -> (w491:waveform(dbl)[])
        n227 = call-poly <vilib>:"DAQmx Write.vi"("task/channels in"=w500, "auto start"=TRUE, "data"=w491) -> ("task out"=w499:refnum<k21>)  [unwired: 10 in, 2 out]
      }
      frame "update 470" {
        n228 = local read "Pulse 470"() -> (w511:bool)
        n229 = local read "Acquire time block"() -> (w506:bool)
        n230 = local read "Begin Experiment"() -> (w508:bool)
        n231 = local read "Run Live"() -> (w507:bool)
        n232 = Build Array(w508, w507, w506) -> (w509:bool[])
        n233 = Or Array Elements(Boolean array=w509) -> (logical OR=w505:bool)
        n234 = case shown="True" w505 {
          tunnel: w511 -> [_ w526]
          tunnel: w516 -> [w519 w521]
          tunnel: [w519 w524] -> w515
          tunnel: w514 -> [w518 w520]
          tunnel: w513 -> [_ w523]
          tunnel: [w518 w522] -> w512
          frame False {
          }
          frame True {
            n235 = local read "470 nm LED control"() -> (w528:dbl)
            n236 = Divide(x=w528, y=20.0) -> (x/y=w525:dbl)
            n237 = case shown="False" w526 {
              tunnel: [w541 w550] -> w524
              tunnel: w525 -> [w540 w559]
              tunnel: w521 -> [w537 w551]
              tunnel: w523 -> [_ w558]
              tunnel: [w529 w542] -> w522
              tunnel: w520 -> [w532 w545]
              frame False {
                n238 = Build Array(w540) -> (w539:dbl[])
                n239 = Bundle By Name("Y"=w539) -> (w538:waveform(dbl))  [unwired: 1 in]
                n240 = Index Array(array=w532, index=1) -> (element=w533:waveform(dbl))
                n241 = call "create single value wavelength of desired length.vi"("waveform (with desired single value)"=w538, "waveform in (for length)"=w533) -> ("output waveform"=w530:waveform(dbl))  [unwired: 9 in]
                n242 = Replace Array Subset(array=w532, new element=w530, index=0) -> (w529:waveform(dbl)[])
                n243 = call <vilib>:"DAQmx Stop Task.vi"("task/channels in"=w537) -> ("task out"=w535:refnum<k21>)  [unwired: 13 in, 1 out]
                n244 = call-poly <vilib>:"DAQmx Write.vi"("task/channels in"=w535, "auto start"=TRUE, "data"=w529) -> ("task out"=w541:refnum<k21>)  [unwired: 10 in, 2 out]
              }
              frame True {
                # "necessary for pulsing to work"
                n245 = To Double Precision Float(number=w558) -> (double precision float=w557:dbl)
                n246 = Index Array(array=w545, index=1) -> (element=w543:waveform(dbl))
                n247 = Unbundle By Name(w543) -> ("Y"=w555:dbl[])
                n248 = property class="DAQmx Timing"(reference=w551) -> (reference out=w547:refnum<k21>, "SampClk.Rate"=w549:dbl)  [unwired: 1 in, 1 out]
                n249 = Index Array(array=w555, index=0) -> (element=w553:dbl)
                n250 = Divide(x="Pulse Duty Cycle", y=100.0) -> (x/y=w556:dbl)
                n251 = Bundle By Name(cluster=T8 {"voltage"=0.0, "frequency"=0.0, "duty cycle"=0.0, "sample rate"=1000.0} ("488 nm channel parameters"), "voltage"=w559, "frequency"=w557, "duty cycle"=w556, "sample rate"=w549) -> (w552:T8)
                n252 = call <vilib>:"DAQmx Stop Task.vi"("task/channels in"=w547) -> ("task out"=w546:refnum<k21>)  [unwired: 13 in, 1 out]
                n253 = call "pulse 488 and steady 594.vi"("594 amplitude"=w553, "488 nm channel parameters"=w552) -> ("waveforms out"=w542:waveform(dbl)[])  [unwired: 9 in]
                n254 = call-poly <vilib>:"DAQmx Write.vi"("task/channels in"=w546, "auto start"=TRUE, "data"=w542) -> ("task out"=w550:refnum<k21>)  [unwired: 10 in, 2 out]
              }
            }
          }
        }
      }
      frame Default {
      }
      frame "Exit" {
      }
    }
    n255 = Send Notification(notification=w167, notifier=w174) -> (notifier out=w175:refnum<notifier>)  [unwired: 1 in, 1 out]
  }
  n256 = while {
    shift-right: [w578] -> w14
    shift-left: w15 -> [w579]
    tunnel: w3 -> [w577]
    tunnel: w4 -> [w574]
    tunnel: w12 -> [w576]
    tunnel: w13 -> [w575]
    tunnel: w11 -> [_]
    tunnel: w10 -> [_]
    tunnel: w9 -> [w572]
    stop <- w573 stop-if-true
    # "UI Events Handler"
    n257 = event shown="[2] \"Acquire time block\": Value Change" {
      selector: w579 -> [_ _ _ _ _ _ _ _ _ _ _]
      dyn-events: [_ _ _ _ _ _ _ _ _ _ _] -> w578
      timeout: _ -> [_ _ _ _ _ _ _ _ _ _ _]
      tunnel: w577 -> [w583 w594 w605 w621 w623 w628 _ _ _ _ _]
      tunnel: w576 -> [_ _ _ _ _ _ w631 w635 w639 w642 _]
      tunnel: w575 -> [_ _ _ _ _ _ _ _ _ _ w648]
      tunnel: w574 -> [_ w593 w606 _ _ _ _ _ _ _ _]
      tunnel: [_ _ _ _ _ _ _ _ _ _ TRUE] -> w573
      tunnel: w572 -> [w582 w592 w607 _ _ w627 _ _ _ _ _]
      event "Run Live": Value Change {
        n258 = event-data() -> ()  [unwired: 1 in, 6 out]
        n259 = case shown="True" "Run Live" {
          tunnel: w583 -> [w584 w587]
          frame False {
            n260 = call "Enqueue Message (Single)_TICO behavior.vi"("Message"="Stop run", "Message Queue"=w584) -> ()  [unwired: 8 in, 2 out]
          }
          frame True {
            n261 = call "Enqueue Message (Single)_TICO behavior.vi"("Message"="update 470", "Message Queue"=w587) -> ("dup Message Queue"=w588:refnum<queue>)  [unwired: 8 in, 1 out]
            n262 = call "Enqueue Message (Single)_TICO behavior.vi"("Message"="Run", "Message Queue"=w588) -> ()  [unwired: 8 in, 2 out]
          }
        }
        n263 = call "Enqueue Message (Single)_TICO behavior.vi"("Message Data"="Run Live", "Message"="Run", "Message Queue"=w582) -> ()  [unwired: 7 in, 2 out]
      }
      event "Begin Experiment": Value Change {
        n264 = event-data() -> ()  [unwired: 1 in, 6 out]
        n265 = case shown="True" "Begin Experiment" {
          tunnel: w594 -> [w597 w600]
          tunnel: w593 -> [w596 w602]
          frame False {
            w595 = "Stop experiment" ("Message")
            n266 = call "Enqueue Message (Single)_TICO behavior.vi"("Message"=w595, "Message Queue"=w597) -> ()  [unwired: 8 in, 2 out]
            n267 = call "Enqueue Message (Single)_TICO behavior.vi"("Message"=w595, "Message Queue"=w596) -> ()  [unwired: 8 in, 2 out]
          }
          frame True {
            w599 = "Begin experiment" ("Message")
            n268 = call "Enqueue Message (Single)_TICO behavior.vi"("Message"=w599, "Message Queue"=w600) -> ("dup Message Queue"=w601:refnum<queue>)  [unwired: 8 in, 1 out]
            n269 = call "Enqueue Message (Single)_TICO behavior.vi"("Message"=w599, "Message Queue"=w602) -> ()  [unwired: 8 in, 2 out]
            n270 = call "Enqueue Message (Single)_TICO behavior.vi"("Message"="update 470", "Message Queue"=w601) -> ()  [unwired: 8 in, 2 out]
          }
        }
        n271 = call "Enqueue Message (Single)_TICO behavior.vi"("Message Data"="Begin Experiment", "Message"="Begin experiment", "Message Queue"=w592) -> ()  [unwired: 7 in, 2 out]
      }
      event "Acquire time block": Value Change {
        n272 = local read "Run time"() -> (w604:i32)
        n273 = event-data() -> ()  [unwired: 1 in, 6 out]
        n274 = Not Equal To 0?(x=w604) -> (x != 0?=w603:bool)
        n275 = case shown="True" w603 {
          tunnel: w607 -> [_ w612]
          tunnel: w606 -> [_ w609]
          tunnel: w605 -> [_ w608]
          frame False {
          }
          frame True {
            n276 = case shown="True" "Acquire time block" {
              tunnel: w609 -> [w613 w620]
              tunnel: w608 -> [w614 w618]
              frame False {
                w615 = "Stop block" ("Message")
                n277 = call "Enqueue Message (Single)_TICO behavior.vi"("Message"=w615, "Message Queue"=w614) -> ()  [unwired: 8 in, 2 out]
                n278 = call "Enqueue Message (Single)_TICO behavior.vi"("Message"=w615, "Message Queue"=w613) -> ()  [unwired: 8 in, 2 out]
              }
              frame True {
                w617 = "Acquire block" ("Message")
                n279 = call "Enqueue Message (Single)_TICO behavior.vi"("Message"=w617, "Message Queue"=w618) -> ("dup Message Queue"=w619:refnum<queue>)  [unwired: 8 in, 1 out]
                n280 = call "Enqueue Message (Single)_TICO behavior.vi"("Message"="update 470", "Message Queue"=w619) -> ()  [unwired: 8 in, 2 out]
                n281 = call "Enqueue Message (Single)_TICO behavior.vi"("Message"=w617, "Message Queue"=w620) -> ()  [unwired: 8 in, 2 out]
              }
            }
            n282 = call "Enqueue Message (Single)_TICO behavior.vi"("Message Data"="Acquire time block", "Message"="Acquire block", "Message Queue"=w612) -> ()  [unwired: 7 in, 2 out]
          }
        }
      }
      event "594 nm laser control": Value Change {
        n283 = event-data() -> ()  [unwired: 1 in, 1 out]
        n284 = call "Enqueue Message (Single)_TICO behavior.vi"("Message"="update 594", "Message Queue"=w621) -> ()  [unwired: 8 in, 2 out]
      }
      event "470 nm LED control", "Pulse Duty Cycle": Value Change {
        n285 = event-data() -> ()  [unwired: 1 in, 6 out]
        n286 = call "Enqueue Message (Single)_TICO behavior.vi"("Message"="update 470", "Message Queue"=w623) -> ()  [unwired: 8 in, 2 out]
      }
      event "Pulse 470": Value Change {
        n287 = event-data() -> ("NewVal"=w625:bool)  [unwired: 1 in, 5 out]
        n288 = call "Enqueue Message (Single)_TICO behavior.vi"("Message"="update 470", "Message Queue"=w628) -> ()  [unwired: 8 in, 2 out]
        n289 = call "Enqueue Message (Single)_TICO behavior.vi"("Message Data"=w625, "Message"="pulse 470", "Message Queue"=w627) -> ()  [unwired: 7 in, 2 out]
      }
      event "Connect SLM": Value Change {
        n290 = event-data() -> ()  [unwired: 1 in, 6 out]
        n291 = case shown="True" "Connect SLM" {
          tunnel: w631 -> [_ w633]
          frame False {
          }
          frame True {
            n292 = call "Enqueue Message (Single)_TICO behavior.vi"("Message"="Connect", "Message Queue"=w633) -> ()  [unwired: 8 in, 2 out]
          }
        }
      }
      event "SLM default": Value Change {
        n293 = event-data() -> ()  [unwired: 1 in, 6 out]
        n294 = case shown="True" "SLM default" {
          tunnel: w635 -> [_ w636]
          frame False {
          }
          frame True {
            n295 = call "Enqueue Message (Single)_TICO behavior.vi"("Message"="SLM high", "Message Queue"=w636) -> ()  [unwired: 8 in, 2 out]
          }
        }
      }
      event "Create SLM image": Value Change {
        n296 = event-data() -> ()  [unwired: 1 in, 6 out]
        n297 = case shown="True" "Create SLM image" {
          tunnel: w639 -> [_ w641]
          frame False {
          }
          frame True {
            n298 = call "Enqueue Message (Single)_TICO behavior.vi"("Message"="Create mask", "Message Queue"=w641) -> ()  [unwired: 8 in, 2 out]
          }
        }
      }
      event "Load SLM image": Value Change {
        n299 = event-data() -> ()  [unwired: 1 in, 6 out]
        n300 = case shown="True" "Load SLM image" {
          tunnel: w642 -> [_ w645]
          frame False {
          }
          frame True {
            n301 = call "Enqueue Message (Single)_TICO behavior.vi"("Message"="Load image", "Message Queue"=w645) -> ()  [unwired: 8 in, 2 out]
          }
        }
      }
      event User Event {
        n302 = event-data() -> ()  [unwired: 1 in, 4 out]
        n303 = call "Enqueue Message (Single)_TICO behavior.vi"("Message"="stop", "Message Queue"=w648) -> ()  [unwired: 8 in, 2 out]
      }
    }
  }
  n304 = while {
    tunnel: w4 -> [w657]
    tunnel: w13 -> [_]
    shift-right: [w654] -> _
    shift-left: _ -> [w649]
    shift-right: [w653] -> _
    shift-left: _ -> [w650]
    stop <- w656 stop-if-true
    # "DAQ acquisition loop"
    n305 = call "Dequeue Message_TICO behavior.vi"("Message Queue"=w657) -> ("Message Data"=w655:variant, "Message"=w658:string)  [unwired: 7 in, 2 out]
    n306 = case shown="\"Log exposures\"" w658 {
      tunnel: [_ TRUE _ _ _ _] -> w656
      tunnel: w655 -> [_ _ _ w688 _ _]
      tunnel: [w660 _ w663 w685 _ w694] -> w654
      tunnel: [w659 _ w662 w684 _ w693] -> w653
      tunnel: "File prefix" -> [_ _ w667 _ _ _]
      tunnel: "Save directory" -> [_ _ w664 _ _ _]
      tunnel: w650 -> [w659 _ _ w683 w692 w693]
      tunnel: w649 -> [w660 _ _ w682 w691 w694]
      frame "Initialize" {
      }
      frame "Stop" {
      }
      frame "Acquire experiment" {
        n307 = Concatenate Strings(w667, "_Kinetix.tdms") -> (w671:string)
        n308 = Concatenate Strings(w667, "_Zelux.tdms") -> (w674:string)
        n309 = String To Path(string=w674) -> (path=w673:path)
        n310 = String To Path(string=w671) -> (path=w672:path)
        n311 = Build Path(base path=w664, name or relative path=w672) -> (appended path=w675:path)
        n312 = Build Path(base path=w664, name or relative path=w673) -> (appended path=w670:path)
        n313 = TDMS Open(10:T11."open or create" ("operation (0:open)"), 11:w670) -> (3:w662:refnum<k34>)  [unwired: 5 in, 1 out]
        n314 = TDMS Open(10:T11."open or create" ("operation (0:open)"), 11:w675) -> (3:w663:refnum<k34>)  [unwired: 5 in, 1 out]
      }
      frame "Log exposures" {
        w680 = waveform(dbl) {"t0"=timestamp(0 s since 1904-01-01), "dt"=1.0, "Y"=[]} ("Waveform")
        w686 = 1.0 ("threshold")
        # "save frame log"
        n315 = Build Array(w680, w680) -> (w687:waveform(dbl)[])
        n316 = Variant To Data(type=w687, Variant=w688) -> (data=w681:waveform(dbl)[])  [unwired: 1 in, 1 out]
        n317 = Index Array(array=w681, index #1=0 ("index"), index #2=1 ("index")) -> (element #1=w677:waveform(dbl), element #2=w676:waveform(dbl))
        n318 = call "extract TTL timing data.vi"("threshold"=w686, "Waveform"=w677) -> ("x+y"=w678:timestamp[])  [unwired: 9 in]
        n319 = call "extract TTL timing data.vi"("threshold"=w686, "Waveform"=w676) -> ("x+y"=w679:timestamp[])  [unwired: 9 in]
        n320 = TDMS Write(0:w682, 9:w678) -> (4:w685:refnum<k34>)  [unwired: 4 in, 3 out]
        n321 = TDMS Write(0:w683, 9:w679) -> (4:w684:refnum<k34>)  [unwired: 4 in, 3 out]
      }
      frame "End acquisition" {
        n322 = TDMS Close(11:w692) -> ()  [unwired: 1 in, 2 out]
        n323 = TDMS Close(11:w691) -> ()  [unwired: 1 in, 2 out]
      }
      frame Default {
      }
    }
  }
  n324 = Unregister For Events(event registration refnum=w14) -> ()  [unwired: 1 in, 1 out]
  n325 = call "Obtain Message Queue_TICO behavior.vi"() -> ("Message Queue"=w2:refnum<queue>)  [unwired: 10 in, 1 out]
  n326 = while {
    tunnel: w9 -> [w697]
    stop <- w695 stop-if-true
    # "UI Display Loop (can switch this to become message handler)"
    n327 = call "Dequeue Message_TICO behavior.vi"("Message Queue"=w697) -> ("Message Data"=w696:variant, "Message"=w698:string)  [unwired: 7 in, 2 out]
    n328 = case shown="\"Initialize\"" w698 {
      tunnel: w696 -> [_ w710 w719 w731 w742 _ _]
      tunnel: [_ _ _ _ _ _ TRUE] -> w695
      frame "Initialize" {
        w700 = FALSE ("Run Live")
        w701 = T6."Enabled" ("Disabled")
        n329 = property on="Pulse Duty Cycle" class="DigNum (strict)"("DisabledEnum"=T6."Disabled and Grayed Out" ("Disabled")) -> ()  [unwired: 2 in, 2 out]
        n330 = property on="Trial progess slide" class="Slide (strict)"("Visible"=FALSE) -> ()  [unwired: 2 in, 2 out]
        n331 = property on="Run Live" class="Bool (strict)"("Caption.Text"="Run live", "DisabledEnum"=w701, "Value"=w700) -> ()  [unwired: 2 in, 2 out]
        n332 = property on="Begin Experiment" class="Bool (strict)"("Caption.Text"="Begin experiment", "DisabledEnum"=w701, "Value"=w700) -> ()  [unwired: 2 in, 2 out]
        n333 = property on="Acquire time block" class="Bool (strict)"("Caption.Text"="Acquire time block", "DisabledEnum"=w701, "Value"=w700) -> ()  [unwired: 2 in, 2 out]
        n334 = property on="Pulse 470" class="Bool (strict)"("Value"=FALSE ("Pulse 470")) -> ()  [unwired: 2 in, 2 out]
      }
      frame "Run" {
        n335 = Variant To Data(type=TRUE, Variant=w710) -> (data=w708:bool)  [unwired: 1 in, 1 out]
        n336 = Boolean To (0,1)(Boolean=w708) -> (0, 1=w712:i16)
        n337 = case shown="False" w708 {
          tunnel: ["Run live" "End live"] -> w711
          frame False {
          }
          frame True {
          }
        }
        n338 = property on="Run Live" class="Bool (strict)"("Value"=w708) -> ()  [unwired: 2 in, 2 out]
        n339 = Multiply(x=w712, y=2.0) -> (x*y=w707:dbl)
        n340 = property on="Run Live" class="Bool (strict)"("Caption.Text"=w711) -> ()  [unwired: 2 in, 2 out]
        n341 = property on="Acquire time block" class="Bool (strict)"("DisabledEnum"=w707) -> ()  [unwired: 2 in, 2 out]
        n342 = property on="Begin Experiment" class="Bool (strict)"("DisabledEnum"=w707) -> ()  [unwired: 2 in, 2 out]
      }
      frame "Begin experiment" {
        n343 = Variant To Data(type=TRUE, Variant=w719) -> (data=w717:bool)  [unwired: 1 in, 1 out]
        n344 = Boolean To (0,1)(Boolean=w717) -> (0, 1=w722:i16)
        n345 = case shown="False" w717 {
          tunnel: ["Begin experiment" "End experiment"] -> w721
          frame False {
          }
          frame True {
          }
        }
        n346 = property on="Begin Experiment" class="Bool (strict)"("Value"=w717) -> ()  [unwired: 2 in, 2 out]
        n347 = Multiply(x=w722, y=2.0) -> (x*y=w718:dbl)
        n348 = property on="Trial progess slide" class="Slide (strict)"("Visible"=w717, "Value"=u8 0 ("Trial progess slide")) -> ()  [unwired: 2 in, 2 out]
        n349 = property on="Begin Experiment" class="Bool (strict)"("Caption.Text"=w721) -> ()  [unwired: 2 in, 2 out]
        n350 = property on="Acquire time block" class="Bool (strict)"("DisabledEnum"=w718) -> ()  [unwired: 2 in, 2 out]
        n351 = property on="Run Live" class="Bool (strict)"("DisabledEnum"=w718) -> ()  [unwired: 2 in, 2 out]
      }
      frame "Acquire block" {
        n352 = Variant To Data(type=TRUE, Variant=w731) -> (data=w730:bool)  [unwired: 1 in, 1 out]
        n353 = Boolean To (0,1)(Boolean=w730) -> (0, 1=w728:i16)
        n354 = property on="Acquire time block" class="Bool (strict)"("Value"=w730) -> ()  [unwired: 2 in, 2 out]
        n355 = case shown="False" w730 {
          tunnel: ["Acquire time block" "End acquisition"] -> w733
          frame False {
          }
          frame True {
          }
        }
        n356 = Multiply(x=w728, y=2.0) -> (x*y=w729:dbl)
        n357 = Multiply(x=w728, y=i16 1) -> (x*y=w726:i16)
        n358 = property on="Acquire time block" class="Bool (strict)"("Caption.Text"=w733) -> ()  [unwired: 2 in, 2 out]
        n359 = property on="Begin Experiment" class="Bool (strict)"("DisabledEnum"=w729) -> ()  [unwired: 2 in, 2 out]
        n360 = property on="Run time" class="DigNum (strict)"("DisabledEnum"=w726) -> ()  [unwired: 2 in, 2 out]
        n361 = property on="Run Live" class="Bool (strict)"("DisabledEnum"=w729) -> ()  [unwired: 2 in, 2 out]
      }
      frame "Pulse 470" {
        n362 = Variant To Data(type=TRUE, Variant=w742) -> (data=w738:bool)  [unwired: 1 in, 1 out]
        n363 = Not(x=w738) -> (.not. x?=w737:bool)
        n364 = Boolean To (0,1)(Boolean=w737) -> (0, 1=w740:i16)
        n365 = Multiply(x=w740, y=2.0) -> (x*y=w739:dbl)
        n366 = property on="Pulse Duty Cycle" class="DigNum (strict)"("DisabledEnum"=w739) -> ()  [unwired: 2 in, 2 out]
      }
      frame Default {
      }
      frame "Exit" {
      }
    }
  }
  n367 = Obtain Notifier(notification data type=variant ("element data type")) -> ()  [unwired: 3 in, 3 out]
  n368 = while {
    tunnel: w10 -> [_]
    tunnel: w13 -> [_]
    shift-right: [w754] -> _
    shift-left: _ -> [w750]
    shift-right: [w752] -> _
    shift-left: _ -> [w749]
    shift-right: [w751] -> _
    shift-left: _ -> [w748]
    shift-right: [w753] -> _
    shift-left: _ -> [w747]
    tunnel: w2 -> [w745]
    stop <- TRUE stop-if-true
    # "PVCam loop"
    n369 = case shown="Default" "" {
      tunnel: [w759 w763 w769 w773 w779] -> w754
      tunnel: [w758 w760 w768 w772 w778] -> w752
      tunnel: [w757 w761 w767 w771 w777] -> w751
      tunnel: [w756 w762 w766 w770 w776] -> w753
      tunnel: w750 -> [w759 w763 w769 _ w779]
      tunnel: w749 -> [w758 w760 w768 _ w778]
      tunnel: w748 -> [w757 w761 w767 _ w777]
      tunnel: w747 -> [w756 w762 w766 _ w776]
      tunnel: w745 -> [_ _ w765 _ _]
      frame "Initialize" {
      }
      frame "Run" {
        # "start"
      }
      frame "Acquire block" {
        n370 = call-poly "Enqueue Message_TICO behavior.vi"("Message"="save images", "Message Queue"=w765) -> ()  [unwired: 8 in, 2 out]
      }
      frame "Connect Kinetix" {
        n371 = call "PV_setup.vi"() -> ("error out"=w771:errorcluster, "Camera out"=w772:refnum<class "Camera.lvclass">, "Camera Description"=w774:T12, "Camera 0 Name"=w775:string, "PVCAM Out"=w770:refnum<class "PVCAM.lvclass">)  [unwired: 7 in]
        n372 = Bundle("Camera 0 Name"=w775, "Camera Description"=w774) -> (w773:T13)  [unwired: 1 in]
      }
      frame Default {
      }
    }
  }
  n373 = Release Notifier(notifier=w7) -> ()  [unwired: 2 in, 3 out]
  n374 = while {
    tunnel: w3 -> [w781]
    tunnel: w6 -> [w783]
    stop <- FALSE stop-if-true
    # "Time blocked run"
    n375 = Wait on Notification(notifier=w783) -> (notification=w782:bool)  [unwired: 3 in, 3 out]
    n376 = flat-sequence {
      tunnel: w782 -> [w786]
      tunnel: [w785] -> w780
      tunnel: w781 -> [w792]
      tunnel: w780 -> [w791]
      frame #0 {
        n377 = case shown="True" w786 {
          tunnel: [_ TRUE] -> w785
          frame False {
          }
          frame True {
            n378 = Multiply(x="Run time", y=1000) -> (x*y=w788:i32)
            n379 = Wait (ms)(milliseconds to wait=w788) -> ()  [unwired: 1 out]
          }
        }
      }
      frame #1 {
        n380 = case shown="True" w791 {
          tunnel: w792 -> [_ w793]
          frame False {
          }
          frame True {
            n381 = call "Enqueue Message (Single)_TICO behavior.vi"("Message"="Stop run", "Message Queue"=w793) -> ()  [unwired: 8 in, 2 out]
          }
        }
      }
    }
  }
  n382 = while {
    shift-right: [w803] -> _
    shift-left: _ -> [w799]
    shift-right: [w801] -> _
    shift-left: _ -> [w798]
    shift-right: [w800] -> _
    shift-left: _ -> [w797]
    shift-right: [w802] -> _
    shift-left: _ -> [w796]
    stop <- TRUE stop-if-true
    # "PVCam acquire loop"
    n383 = case shown="\"Run\"" "" {
      tunnel: [w808 w812 w816 w820 w826] -> w803
      tunnel: [w807 w809 w815 w819 w825] -> w801
      tunnel: [w806 w810 w814 w818 w824] -> w800
      tunnel: [w805 w811 w813 w817 w823] -> w802
      tunnel: w799 -> [w808 w812 w816 _ w826]
      tunnel: w798 -> [w807 w809 w815 _ w825]
      tunnel: w797 -> [w806 w810 w814 _ w824]
      tunnel: w796 -> [w805 w811 w813 _ w823]
      frame "Initialize" {
      }
      frame "Run" {
        # "start"
      }
      frame "Acquire block" {
      }
      frame "Connect Kinetix" {
        n384 = call "PV_setup.vi"() -> ("error out"=w818:errorcluster, "Camera out"=w819:refnum<class "Camera.lvclass">, "Camera Description"=w821:T12, "Camera 0 Name"=w822:string, "PVCAM Out"=w817:refnum<class "PVCAM.lvclass">)  [unwired: 7 in]
        n385 = Bundle("Camera 0 Name"=w822, "Camera Description"=w821) -> (w820:T13)  [unwired: 1 in]
      }
      frame Default {
      }
    }
  }
